vi "STD Filter.vi"(5 "Cal STD in":string[][](array[string]), 7 "STD select":T1, 8 "문자열(option, STD)":string, 9 "Condition":string[][](array[string]), 11 "값(option)":string) -> (0 "제외 DATA 출력":string[][](array[string]), 1 "Cal STD out":string[][](array[string]), 2 "비어있음?":bool, 3 "DATA 출력":string[][](array[string]), 4 "문자열(option, STD)":string)   [LabVIEW 2020]
uses:
  Controls/Cmd_STD select.ctl
  Public/Polymorph/Data Class_2D Str.vi
  Public/Polymorph/Sort_2D Str.vi
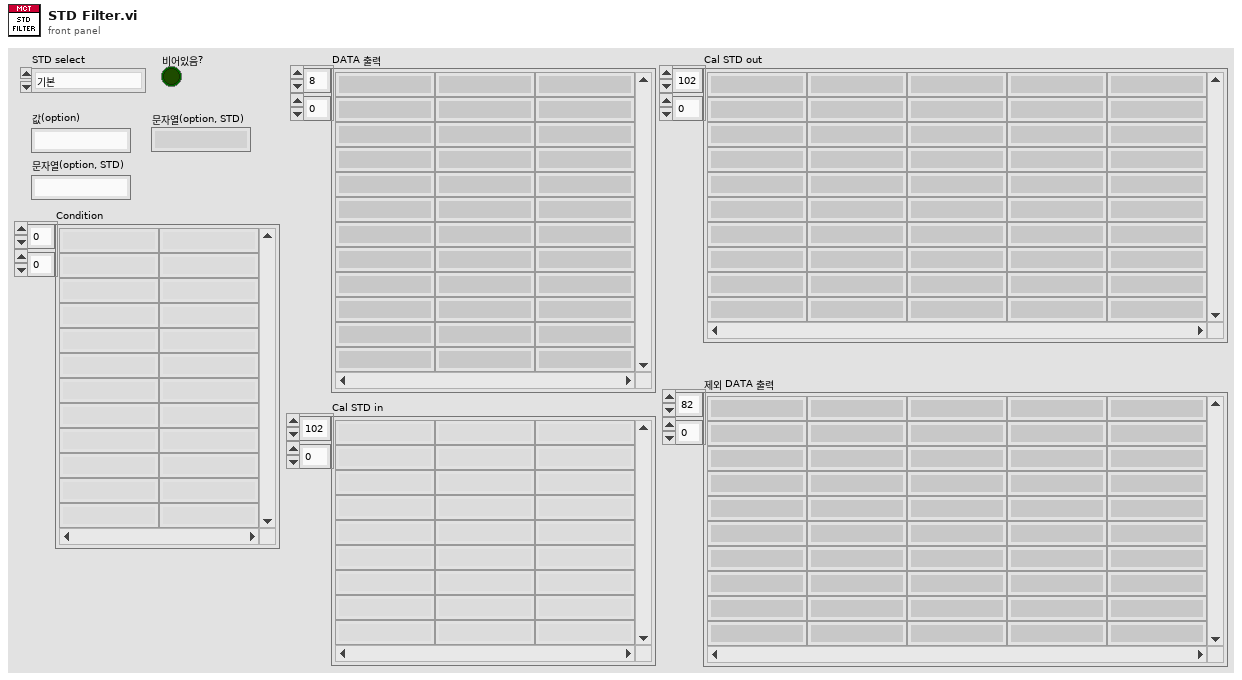
[diagram p1: front panel]
types:
  T1 = typedef "Cmd_STD select.ctl" = enum16{"기본", "DMM", "Electronic Micrometer", "Fine Angle Generator", "Measuring Projector", "Precision Square", "Power Supply", "Ring Gauge", "Straight Edge", "Thermo-Hygrometer", "Calibrator"}
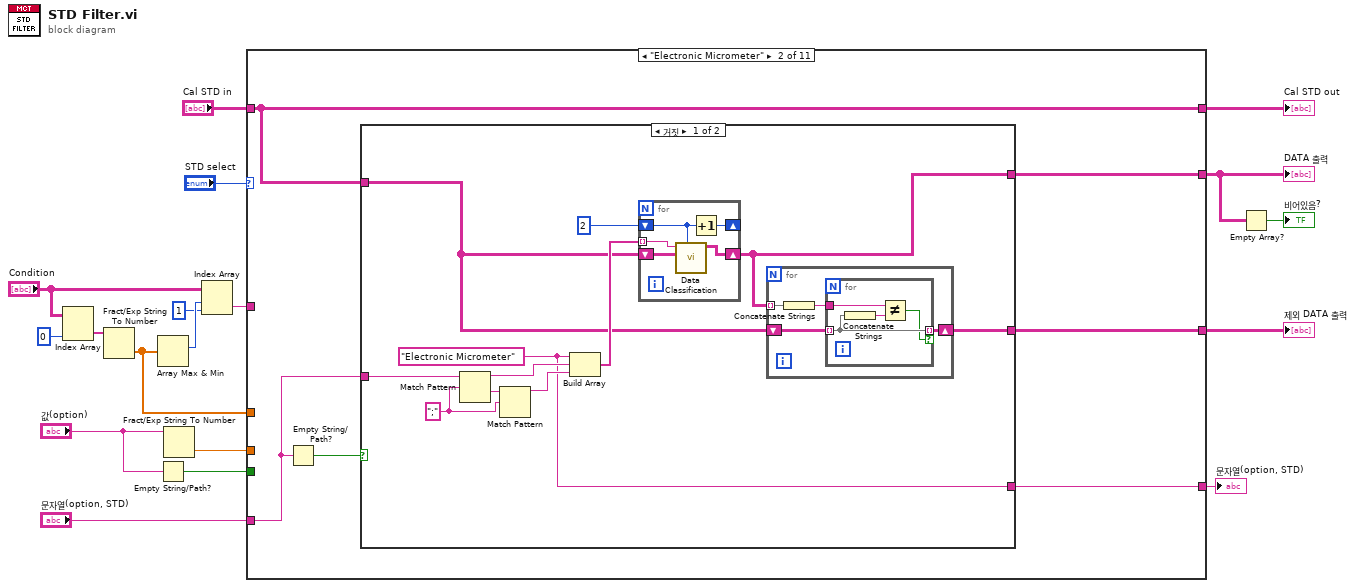
[diagram p0: block diagram]
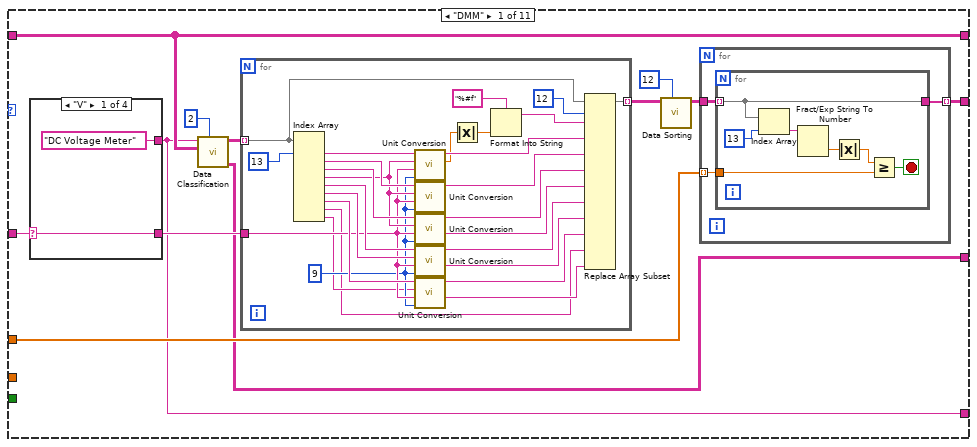
[diagram p2: hidden frame]
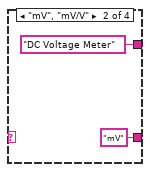
[diagram p3: hidden frame]
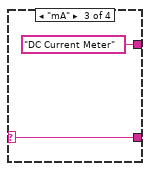
[diagram p4: hidden frame]
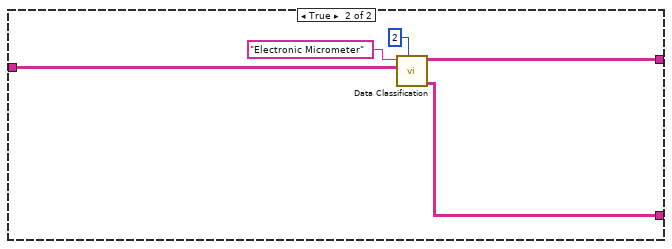
[diagram p6: hidden frame]
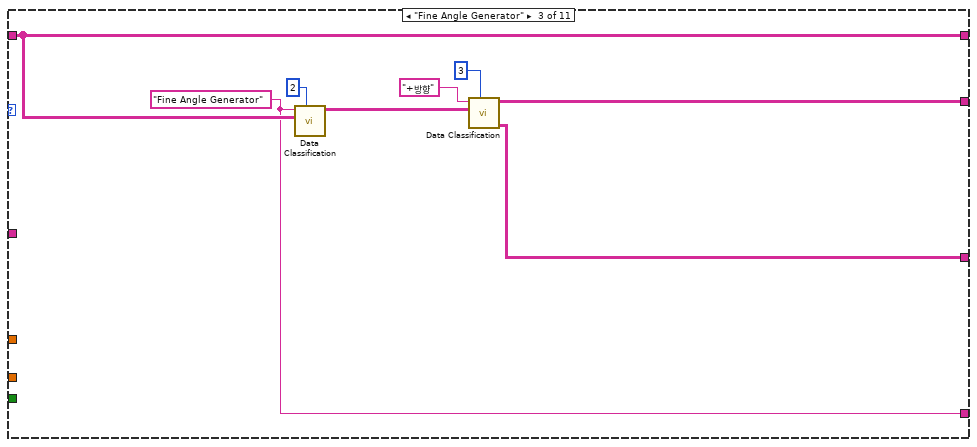
[diagram p7: hidden frame]
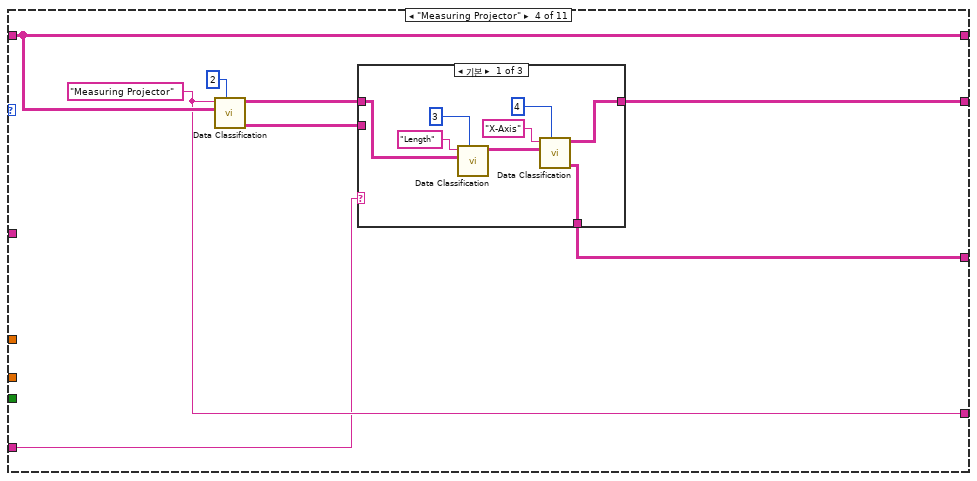
[diagram p8: hidden frame]
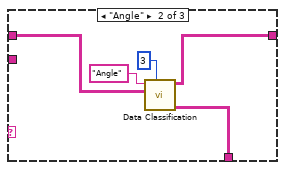
[diagram p9: hidden frame]
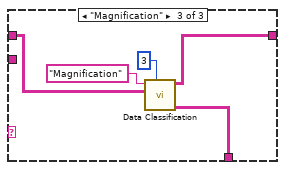
[diagram p10: hidden frame]
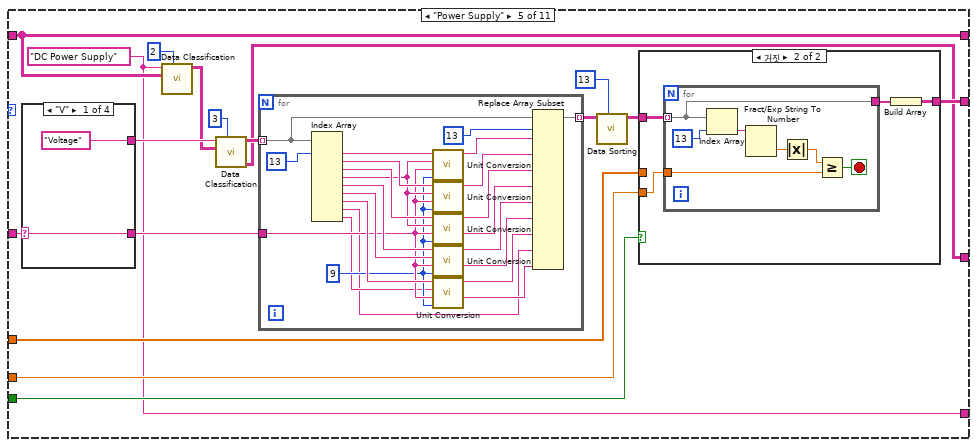
[diagram p11: hidden frame]
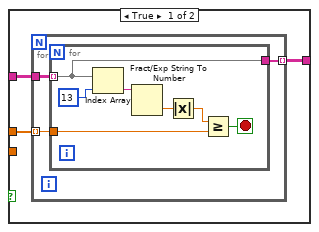
[diagram p12: hidden frame]
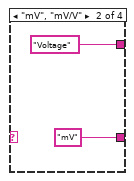
[diagram p13: hidden frame]
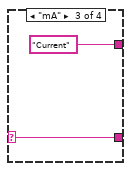
[diagram p14: hidden frame]
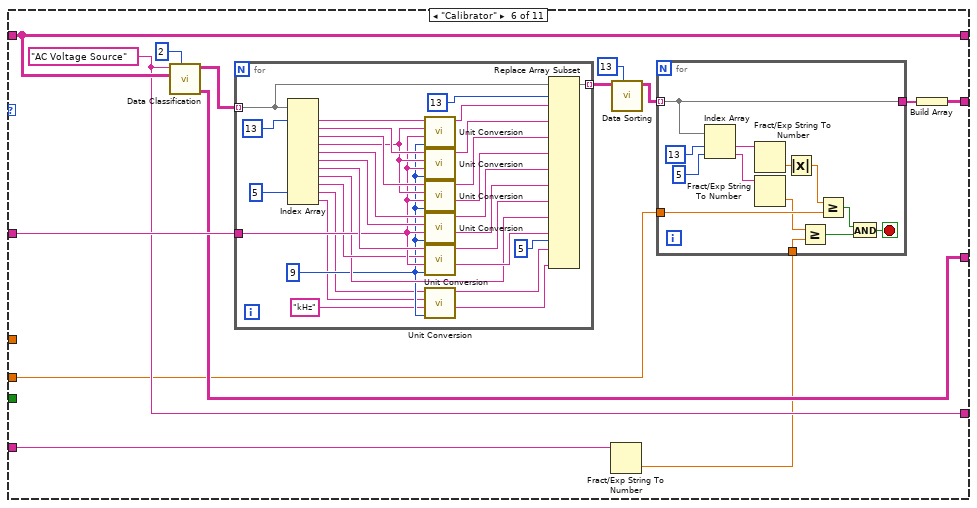
[diagram p16: hidden frame]
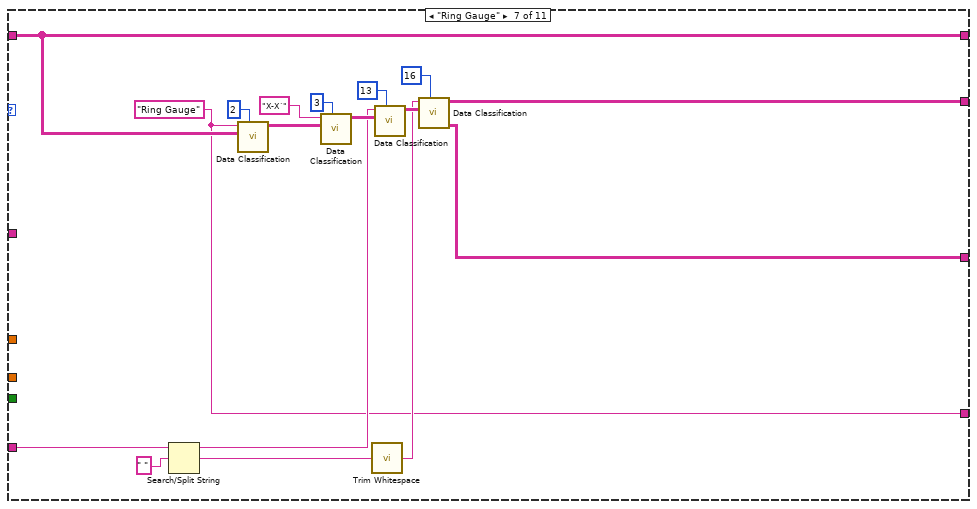
[diagram p17: hidden frame]
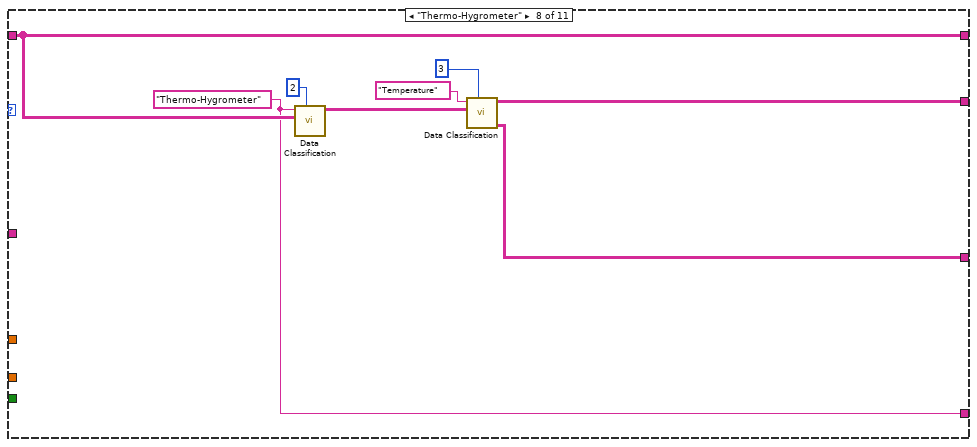
[diagram p18: hidden frame]
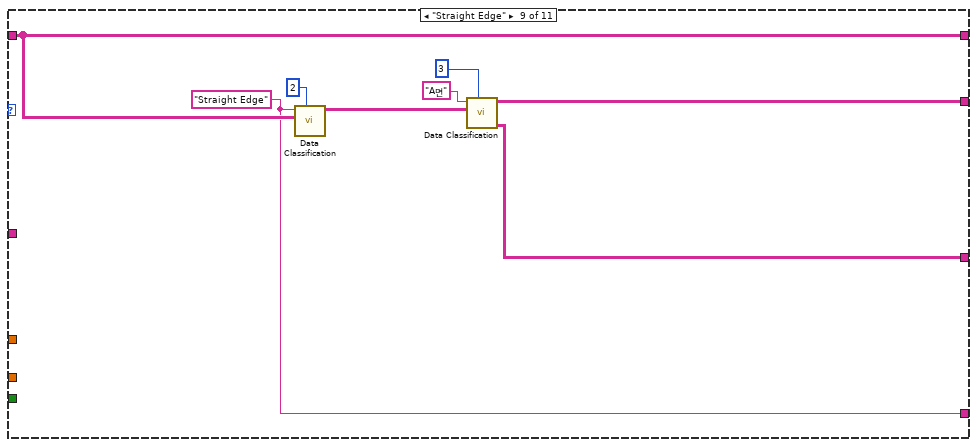
[diagram p19: hidden frame]
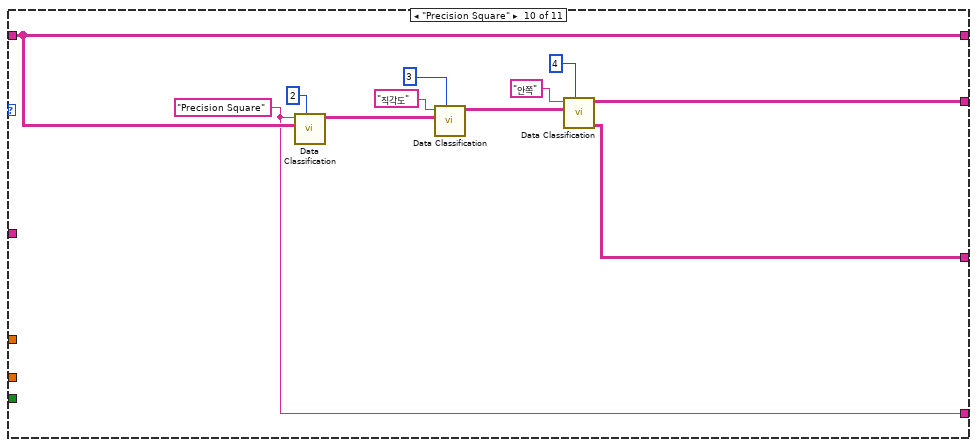
[diagram p20: hidden frame]
diagram:
  n1 = Index Array(array="Condition", index (col)=0 ("비활성화된 인덱스 (열)")) -> (element=w16:string[])  [unwired: 1 in]
  n2 = Fract/Exp String To Number(string=w16) -> (number=w11:dbl[])  [unwired: 3 in, 1 out]
  n3 = Array Max & Min(array=w11) -> (max index (indices)=w15:i32)  [unwired: 3 out]
  n4 = Empty String/Path?(string/path="값(option)") -> (empty?=w8:bool)
  n5 = Fract/Exp String To Number(string="값(option)") -> (number=w10:dbl)  [unwired: 3 in, 1 out]
  n6 = Index Array(array="Condition", index (row)=w15, index (col)=1 ("비활성화된 인덱스 (열)")) -> (element=w12:string)
  n7 = case shown="\"Electronic Micrometer\"" "STD select" {
    tunnel: w12 -> [w30 _ _ _ w159 w226 _ _ _ _ _]
    tunnel: "Cal STD in" -> [w21 w79 w115 w123 w145 w219 w278 w293 w301 w312 w317]
    tunnel: [w23 w78 w111 w121 w151 w213 w277 w289 w297 w303 w316] -> w4
    tunnel: w11 -> [w24 _ _ _ w150 _ _ _ _ _ _]
    tunnel: w10 -> [_ _ _ _ w148 w214 _ _ _ _ _]
    tunnel: w8 -> [_ _ _ _ w149 _ _ _ _ _ _]
    tunnel: [w21 w79 w115 w123 w145 w219 w278 w293 w301 w312 w317] -> w7
    tunnel: "문자열(option, STD)" -> [_ w75 _ w118 _ w216 w274 _ _ _ w315]
    tunnel: [w20 w77 w110 w120 w144 w217 w271 w288 w296 w304 w314] -> w2
    tunnel: [w19 w76 w109 w119 w143 w218 w270 w287 w295 w308 w315] -> w1
    frame "DMM" {
      n8 = case shown="\"V\"" w30 {
        selector: w30 -> [w41 _ w45 _]
        tunnel: ["DC Voltage Meter" "DC Voltage Meter" "DC Current Meter" _] -> w19
        tunnel: [w41 "mV" w45 _] -> w29
        frame "V" {
        }
        frame "mV", "mV/V" {
        }
        frame "mA" {
        }
        frame Default {
        }
      }
      n9 = call-poly "Data Classification.vi"("인덱스"=2, "DATA 입력"=w21, "검색 문자열"=w19) -> ("제외 DATA 출력"=w20:string[][], "DATA 출력"=w22:string[][])  [unwired: 4 in, 3 out]
      n10 = for {
        tunnel: w22 -> [w71] mode=indexing
        tunnel: w29 -> [w57]
        tunnel: [w69] -> w28 mode=indexing
        w56 = 9 ("소수점 자리수")
        n11 = Index Array(array=w71, index #1=13 ("인덱스")) -> (element #1=w72:string, element #2=w68:string, element #3=w67:string, element #4=w66:string, element #5=w62:string, element #6=w61:string, element #7=w58:string, element #8=w52:string, element #9=w54:string)  [unwired: 8 in]
        n12 = call "Unit Conversion.vi"("소수점 자리수"=w56, "환산단위"=w57, "입력단위"=w66, "입력값"=w72) -> ("환산값 (DBL)"=w50:dbl, "환산값 (string)"=w70:string)  [unwired: 2 in, 4 out]
        n13 = call "Unit Conversion.vi"("소수점 자리수"=w56, "환산단위"=w57, "입력단위"=w66, "입력값"=w68) -> ("환산값 (string)"=w65:string)  [unwired: 2 in, 5 out]
        n14 = call "Unit Conversion.vi"("소수점 자리수"=w56, "환산단위"=w57, "입력단위"=w66, "입력값"=w67) -> ("환산단위"=w63:string, "환산값 (string)"=w64:string)  [unwired: 2 in, 4 out]
        n15 = call "Unit Conversion.vi"("소수점 자리수"=w56, "환산단위"=w57, "입력단위"=w61, "입력값"=w62) -> ("환산단위"=w59:string, "환산값 (string)"=w60:string)  [unwired: 2 in, 4 out]
        n16 = call "Unit Conversion.vi"("소수점 자리수"=w56, "환산단위"=w57, "입력단위"=w54, "입력값"=w58) -> ("환산단위"=w53:string, "환산값 (string)"=w55:string)  [unwired: 2 in, 4 out]
        n17 = Absolute Value(x=w50) -> (abs(x)=w47:dbl)
        n18 = Format Into String(format string="%#f" ("포맷 문자열"), w47) -> (resulting string=w49:string)  [unwired: 2 in, 1 out]
        n19 = Replace Array Subset(array=w71, new element #1=w49, index #1=12 ("인덱스"), new element #2=w70, new element #3=w65, new element #4=w64, new element #5=w63, new element #6=w60, new element #7=w59, new element #8=w55, new element #9=w52, new element #10=w53) -> (w69:string[])  [unwired: 9 in]
      }
      n20 = call-poly "Data Sorting.vi"("기준열"=u16 12, "Data in"=w28) -> ("Data out"=w25:string[][])  [unwired: 8 in, 1 out]
      n21 = for {
        tunnel: w25 -> [w33]
        tunnel: w24 -> [w32] mode=indexing
        tunnel: [w31] -> w23 mode=indexing
        n22 = for {
          tunnel: w33 -> [w34] mode=indexing
          tunnel: w32 -> [w37]
          tunnel: [w34] -> w31
          stop <- w35 stop-if-true
          n23 = Index Array(array=w34, index=13 ("인덱스")) -> (element=w39:string)
          n24 = Fract/Exp String To Number(string=w39) -> (number=w38:dbl)  [unwired: 3 in, 1 out]
          n25 = Absolute Value(x=w38) -> (abs(x)=w36:dbl)
          n26 = Greater Or Equal?(x=w36, y=w37) -> (x >= y?=w35:bool)
        }
      }
    }
    frame "Electronic Micrometer" {
      n27 = Empty String/Path?(string/path=w75) -> (empty?=w74:bool)
      n28 = case shown="거짓" w74 {
        tunnel: w79 -> [w81 w106]
        tunnel: [w82 w105] -> w78
        tunnel: [w80 w104] -> w77
        tunnel: [w84 _] -> w76
        tunnel: w75 -> [w83 _]
        frame False {
          w84 = "Electronic Micrometer"
          w90 = ";" ("정규식")
          n29 = Match Pattern(string=w83, regular expression=w90) -> (before substring=w85:string, after substring=w88:string)  [unwired: 1 in, 2 out]
          n30 = Match Pattern(string=w88, regular expression=w90) -> (before substring=w89:string)  [unwired: 1 in, 3 out]
          n31 = Build Array(w84, w85, w89) -> (w86:string[])
          n32 = for {
            shift-right: [w102] -> w82
            shift-left: w81 -> [w103]
            tunnel: w86 -> [w100] mode=indexing
            shift-right: [w101] -> _
            shift-left: 2 ("비활성화된 인덱스 (열)") -> [w99]
            n33 = call-poly "Data Classification.vi"("인덱스"=w99, "DATA 입력"=w103, "검색 문자열"=w100) -> ("DATA 출력"=w102:string[][])  [unwired: 4 in, 4 out]
            n34 = Increment(x=w99) -> (x+1=w101:i32)
          }
          n35 = for {
            tunnel: w82 -> [w94] mode=indexing
            shift-right: [w91] -> w80
            shift-left: w81 -> [w93]
            n36 = Concatenate Strings(w94) -> (w92:string)
            n37 = for {
              tunnel: w93 -> [w96] mode=indexing
              tunnel: w92 -> [w97]
              tunnel: [w96] -> w91 mode=indexing if=w95
              n38 = Concatenate Strings(w96) -> (w98:string)
              n39 = Not Equal?(x=w97, y=w98) -> (x != y?=w95:bool)
            }
          }
        }
        frame True {
          n40 = call-poly "Data Classification.vi"("인덱스"=2, "DATA 입력"=w106, "검색 문자열"="Electronic Micrometer") -> ("제외 DATA 출력"=w104:string[][], "DATA 출력"=w105:string[][])  [unwired: 4 in, 3 out]
        }
      }
    }
    frame "Fine Angle Generator" {
      w109 = "Fine Angle Generator" ("검색 문자열")
      n41 = call-poly "Data Classification.vi"("인덱스"=2, "DATA 입력"=w115, "검색 문자열"=w109) -> ("DATA 출력"=w112:string[][])  [unwired: 4 in, 4 out]
      n42 = call-poly "Data Classification.vi"("인덱스"=3, "DATA 입력"=w112, "검색 문자열"="+방향") -> ("제외 DATA 출력"=w110:string[][], "DATA 출력"=w111:string[][])  [unwired: 4 in, 3 out]
    }
    frame "Measuring Projector" {
      w119 = "Measuring Projector" ("검색 문자열")
      n43 = call-poly "Data Classification.vi"("인덱스"=2, "DATA 입력"=w123, "검색 문자열"=w119) -> ("제외 DATA 출력"=w117:string[][], "DATA 출력"=w122:string[][])  [unwired: 4 in, 3 out]
      n44 = case shown="기본" w118 {
        tunnel: w122 -> [w127 w135 w140]
        tunnel: [w126 w134 w139] -> w121
        tunnel: [w125 w133 w138] -> w120
        tunnel: w117 -> [_ _ _]
        frame Default {
          n45 = call-poly "Data Classification.vi"("인덱스"=3, "DATA 입력"=w127, "검색 문자열"="Length") -> ("DATA 출력"=w132:string[][])  [unwired: 4 in, 4 out]
          n46 = call-poly "Data Classification.vi"("인덱스"=4, "DATA 입력"=w132, "검색 문자열"="X-Axis") -> ("제외 DATA 출력"=w125:string[][], "DATA 출력"=w126:string[][])  [unwired: 4 in, 3 out]
        }
        frame "Angle" {
          n47 = call-poly "Data Classification.vi"("인덱스"=3, "DATA 입력"=w135, "검색 문자열"="Angle") -> ("제외 DATA 출력"=w133:string[][], "DATA 출력"=w134:string[][])  [unwired: 4 in, 3 out]
        }
        frame "Magnification" {
          n48 = call-poly "Data Classification.vi"("인덱스"=3, "DATA 입력"=w140, "검색 문자열"="Magnification") -> ("제외 DATA 출력"=w138:string[][], "DATA 출력"=w139:string[][])  [unwired: 4 in, 3 out]
        }
      }
    }
    frame "Power Supply" {
      w143 = "DC Power Supply" ("검색 문자열")
      n49 = case shown="\"V\"" w159 {
        selector: w159 -> [w184 _ w188 _]
        tunnel: ["Voltage" "Voltage" "Current" _] -> w158
        tunnel: [w184 "mV" w188 _] -> w156
        frame "V" {
        }
        frame "mV", "mV/V" {
        }
        frame "mA" {
        }
        frame Default {
        }
      }
      n50 = call-poly "Data Classification.vi"("인덱스"=2, "DATA 입력"=w145, "검색 문자열"=w143) -> ("DATA 출력"=w146:string[][])  [unwired: 4 in, 4 out]
      n51 = call-poly "Data Classification.vi"("인덱스"=3, "DATA 입력"=w146, "검색 문자열"=w158) -> ("제외 DATA 출력"=w144:string[][], "DATA 출력"=w157:string[][])  [unwired: 4 in, 3 out]
      n52 = for {
        tunnel: w157 -> [w210] mode=indexing
        tunnel: w156 -> [w195]
        tunnel: [w207] -> w155 mode=indexing
        w194 = 9 ("소수점 자리수")
        n53 = Index Array(array=w210, index #1=13 ("인덱스")) -> (element #1=w211:string, element #2=w206:string, element #3=w205:string, element #4=w204:string, element #5=w200:string, element #6=w199:string, element #7=w196:string, element #8=w190:string, element #9=w192:string)  [unwired: 8 in]
        n54 = call "Unit Conversion.vi"("소수점 자리수"=w194, "환산단위"=w195, "입력단위"=w204, "입력값"=w211) -> ("환산값 (string)"=w208:string)  [unwired: 2 in, 5 out]
        n55 = call "Unit Conversion.vi"("소수점 자리수"=w194, "환산단위"=w195, "입력단위"=w204, "입력값"=w206) -> ("환산값 (string)"=w203:string)  [unwired: 2 in, 5 out]
        n56 = call "Unit Conversion.vi"("소수점 자리수"=w194, "환산단위"=w195, "입력단위"=w204, "입력값"=w205) -> ("환산단위"=w201:string, "환산값 (string)"=w202:string)  [unwired: 2 in, 4 out]
        n57 = call "Unit Conversion.vi"("소수점 자리수"=w194, "환산단위"=w195, "입력단위"=w199, "입력값"=w200) -> ("환산단위"=w197:string, "환산값 (string)"=w198:string)  [unwired: 2 in, 4 out]
        n58 = call "Unit Conversion.vi"("소수점 자리수"=w194, "환산단위"=w195, "입력단위"=w192, "입력값"=w196) -> ("환산단위"=w191:string, "환산값 (string)"=w193:string)  [unwired: 2 in, 4 out]
        n59 = Replace Array Subset(array=w210, new element #1=w208, index #1=13 ("인덱스"), new element #2=w203, new element #3=w202, new element #4=w201, new element #5=w198, new element #6=w197, new element #7=w193, new element #8=w190, new element #9=w191) -> (w207:string[])  [unwired: 8 in]
      }
      n60 = call-poly "Data Sorting.vi"("기준열"=u16 13, "Data in"=w155) -> ("Data out"=w152:string[][])  [unwired: 8 in, 1 out]
      n61 = case shown="거짓" w149 {
        tunnel: w152 -> [w162 w176]
        tunnel: [w161 w173] -> w151
        tunnel: w150 -> [w160 _]
        tunnel: w148 -> [_ w174]
        frame True {
          n62 = for {
            tunnel: w162 -> [w165]
            tunnel: [w164] -> w161 mode=indexing
            tunnel: w160 -> [w163] mode=indexing
            n63 = for {
              tunnel: w165 -> [w166] mode=indexing
              tunnel: w163 -> [w169]
              tunnel: [w166] -> w164
              stop <- w167 stop-if-true
              n64 = Index Array(array=w166, index=13 ("인덱스")) -> (element=w171:string)
              n65 = Fract/Exp String To Number(string=w171) -> (number=w170:dbl)  [unwired: 3 in, 1 out]
              n66 = Absolute Value(x=w170) -> (abs(x)=w168:dbl)
              n67 = Greater Or Equal?(x=w168, y=w169) -> (x >= y?=w167:bool)
            }
          }
        }
        frame False {
          n68 = for {
            tunnel: w176 -> [w177] mode=indexing
            tunnel: w174 -> [w180]
            tunnel: [w177] -> w175
            stop <- w178 stop-if-true
            n69 = Index Array(array=w177, index=13 ("인덱스")) -> (element=w182:string)
            n70 = Fract/Exp String To Number(string=w182) -> (number=w181:dbl)  [unwired: 3 in, 1 out]
            n71 = Absolute Value(x=w181) -> (abs(x)=w179:dbl)
            n72 = Greater Or Equal?(x=w179, y=w180) -> (x >= y?=w178:bool)
          }
          n73 = Build Array(w175) -> (w173:string[][])
        }
      }
    }
    frame "Calibrator" {
      w218 = "AC Voltage Source" ("검색 문자열")
      n74 = call-poly "Data Classification.vi"("인덱스"=2, "DATA 입력"=w219, "검색 문자열"=w218) -> ("제외 DATA 출력"=w217:string[][], "DATA 출력"=w220:string[][])  [unwired: 4 in, 3 out]
      n75 = for {
        tunnel: w220 -> [w267] mode=indexing
        tunnel: w226 -> [w252]
        tunnel: [w264] -> w225 mode=indexing
        w246 = 9 ("소수점 자리수")
        n76 = Index Array(array=w267, index #1=13 ("인덱스"), index #10=5 ("인덱스")) -> (element #1=w268:string, element #2=w263:string, element #3=w262:string, element #4=w261:string, element #5=w257:string, element #6=w256:string, element #7=w253:string, element #8=w248:string, element #9=w250:string, element #10=w245:string, element #11=w244:string)  [unwired: 9 in]
        n77 = call "Unit Conversion.vi"("소수점 자리수"=w246, "환산단위"=w252, "입력단위"=w261, "입력값"=w268) -> ("환산값 (string)"=w265:string)  [unwired: 2 in, 5 out]
        n78 = call "Unit Conversion.vi"("소수점 자리수"=w246, "환산단위"=w252, "입력단위"=w261, "입력값"=w263) -> ("환산값 (string)"=w260:string)  [unwired: 2 in, 5 out]
        n79 = call "Unit Conversion.vi"("소수점 자리수"=w246, "환산단위"=w252, "입력단위"=w261, "입력값"=w262) -> ("환산단위"=w258:string, "환산값 (string)"=w259:string)  [unwired: 2 in, 4 out]
        n80 = call "Unit Conversion.vi"("소수점 자리수"=w246, "환산단위"=w252, "입력단위"=w256, "입력값"=w257) -> ("환산단위"=w254:string, "환산값 (string)"=w255:string)  [unwired: 2 in, 4 out]
        n81 = call "Unit Conversion.vi"("소수점 자리수"=w246, "환산단위"=w252, "입력단위"=w250, "입력값"=w253) -> ("환산단위"=w249:string, "환산값 (string)"=w251:string)  [unwired: 2 in, 4 out]
        n82 = call "Unit Conversion.vi"("소수점 자리수"=w246, "환산단위"="kHz", "입력단위"=w244, "입력값"=w245) -> ("환산단위"=w240:string, "환산값 (string)"=w241:string)  [unwired: 2 in, 4 out]
        n83 = Replace Array Subset(array=w267, new element #1=w265, index #1=13 ("인덱스"), new element #2=w260, new element #3=w259, new element #4=w258, new element #5=w255, new element #6=w254, new element #7=w251, new element #8=w248, new element #9=w249, new element #10=w241, index #10=5 ("인덱스"), new element #11=w240) -> (w264:string[])  [unwired: 9 in]
      }
      n84 = Fract/Exp String To Number(string=w216) -> (number=w215:dbl)  [unwired: 3 in, 1 out]
      n85 = call-poly "Data Sorting.vi"("기준열"=u16 13, "Data in"=w225) -> ("Data out"=w223:string[][])  [unwired: 8 in, 1 out]
      n86 = for {
        tunnel: w223 -> [w234] mode=indexing
        tunnel: w214 -> [w236]
        tunnel: [w234] -> w222
        tunnel: w215 -> [w230]
        stop <- w227 stop-if-true
        n87 = Index Array(array=w234, index #1=13 ("인덱스"), index #2=5 ("인덱스")) -> (element #1=w238:string, element #2=w232:string)
        n88 = Fract/Exp String To Number(string=w238) -> (number=w237:dbl)  [unwired: 3 in, 1 out]
        n89 = Fract/Exp String To Number(string=w232) -> (number=w231:dbl)  [unwired: 3 in, 1 out]
        n90 = Absolute Value(x=w237) -> (abs(x)=w235:dbl)
        n91 = Greater Or Equal?(x=w231, y=w230) -> (x >= y?=w228:bool)
        n92 = Greater Or Equal?(x=w235, y=w236) -> (x >= y?=w229:bool)
        n93 = And(x=w229, y=w228) -> (x .and. y?=w227:bool)
      }
      n94 = Build Array(w222) -> (w213:string[][])
    }
    frame "Ring Gauge" {
      w270 = "Ring Gauge"
      n95 = Search/Split String(string=w274, search string/char (-)=" " ("검색 문자열/문자 (-)")) -> (substring before match=w273:string, match + rest of string=w276:string)  [unwired: 1 in, 1 out]
      n96 = call-poly "Data Classification.vi"("인덱스"=2, "DATA 입력"=w278, "검색 문자열"=w270) -> ("DATA 출력"=w281:string[][])  [unwired: 4 in, 4 out]
      n97 = call-poly "Data Classification.vi"("인덱스"=3, "DATA 입력"=w281, "검색 문자열"="X-X´") -> ("DATA 출력"=w284:string[][])  [unwired: 4 in, 4 out]
      n98 = call <vilib>:"Trim Whitespace.vi"("string"=w276) -> ("trimmed string"=w272:string)  [unwired: 1 in]
      n99 = call-poly "Data Classification.vi"("인덱스"=13, "DATA 입력"=w284, "검색 문자열"=w273) -> ("DATA 출력"=w286:string[][])  [unwired: 4 in, 4 out]
      n100 = call-poly "Data Classification.vi"("인덱스"=16, "DATA 입력"=w286, "검색 문자열"=w272) -> ("제외 DATA 출력"=w271:string[][], "DATA 출력"=w277:string[][])  [unwired: 4 in, 3 out]
    }
    frame "Thermo-Hygrometer" {
      w287 = "Thermo-Hygrometer" ("검색 문자열")
      n101 = call-poly "Data Classification.vi"("인덱스"=2, "DATA 입력"=w293, "검색 문자열"=w287) -> ("DATA 출력"=w290:string[][])  [unwired: 4 in, 4 out]
      n102 = call-poly "Data Classification.vi"("인덱스"=3, "DATA 입력"=w290, "검색 문자열"="Temperature") -> ("제외 DATA 출력"=w288:string[][], "DATA 출력"=w289:string[][])  [unwired: 4 in, 3 out]
    }
    frame "Straight Edge" {
      w295 = "Straight Edge" ("검색 문자열")
      n103 = call-poly "Data Classification.vi"("인덱스"=2, "DATA 입력"=w301, "검색 문자열"=w295) -> ("DATA 출력"=w298:string[][])  [unwired: 4 in, 4 out]
      n104 = call-poly "Data Classification.vi"("인덱스"=3, "DATA 입력"=w298, "검색 문자열"="A면") -> ("제외 DATA 출력"=w296:string[][], "DATA 출력"=w297:string[][])  [unwired: 4 in, 3 out]
    }
    frame "Precision Square" {
      w308 = "Precision Square" ("검색 문자열")
      n105 = call-poly "Data Classification.vi"("인덱스"=2, "DATA 입력"=w312, "검색 문자열"=w308) -> ("DATA 출력"=w309:string[][])  [unwired: 4 in, 4 out]
      n106 = call-poly "Data Classification.vi"("인덱스"=3, "DATA 입력"=w309, "검색 문자열"="직각도") -> ("DATA 출력"=w307:string[][])  [unwired: 4 in, 4 out]
      n107 = call-poly "Data Classification.vi"("인덱스"=4, "DATA 입력"=w307, "검색 문자열"="안쪽") -> ("제외 DATA 출력"=w304:string[][], "DATA 출력"=w303:string[][])  [unwired: 4 in, 3 out]
    }
    frame Default {
      # "Angle Gauge Block\nCaliper Tester\nCoating Thickness Specimen\nStep Gauge\nGauge Block\nGauge Block Comparator\nMonochromatic Light Source\nStandard Measuring Machine\nStandard Optical Flat\nSurface Plate\nTape Measure Calibration System\nThread Measuring Wire Gauge\nUltrasonic Thickness Specimen"
      n108 = call-poly "Data Classification.vi"("인덱스"=2, "DATA 입력"=w317, "검색 문자열"=w315) -> ("제외 DATA 출력"=w314:string[][], "DATA 출력"=w316:string[][])  [unwired: 4 in, 3 out]
    }
  }
  "Cal STD out" <- w7
  "DATA 출력" <- w4
  "제외 DATA 출력" <- w2
  "문자열(option, STD)" <- w1
  n109 = Empty Array?(array=w4) -> (empty?=→"비어있음?":bool)
